vi "color.vi"() -> ()   [LabVIEW 2016]
uses:
  <vilib>/NXT/Subs/LVHSConnector.ctl
  <vilib>/NXT/LegoClasses/BrickReference/BrickReference.lvclass
  <vilib>/NXT/Block Support/NXT_InputPort.ctl
  <vilib>/NXT/Subs/ColorSensorColors.ctl
  <vilib>/NXT/Block Support/NXT_OutputPort.ctl
  <vilib>/NXT/Dual Mode Library/Display/drawNumber.vi
  <vilib>/NXT/Dual Mode Library/Sensors/Color_Detector.vi
  <vilib>/NXT/NXTIO Xnodes/NXTIONodeSubVIs/NXTStopMotors.vi
  <vilib>/NXT/NXTIO Xnodes/NXTIONodeSubVIs/NXTMoveMotors.vi
  <vilib>/NXT/NXTIO Xnodes/AddressXNode/NXTIOAddress.xnode
  <vilib>/NXT/NXTIO Xnodes/NXTIOXNode/NXTIO.xnode
panel:
  in  "NXT/EV3":T1
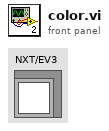
[diagram p1: front panel]
types:
  T1 = typedef "LVHSConnector.ctl" = refnum<class "BrickReference.lvclass">
  T2 = typedef "ColorSensorColors.ctl" = enum16{"No Color", "Black", "Blue", "Green", "Yellow", "Red", "White", "Brown"}
  T3 = typedef "NXT_OutputPort.ctl" = u8
  T4 = typedef "NXT_InputPort.ctl" = u32
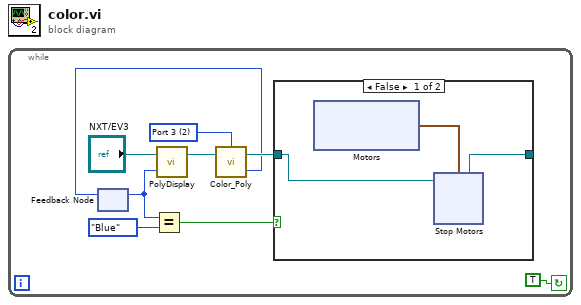
[diagram p0: block diagram]
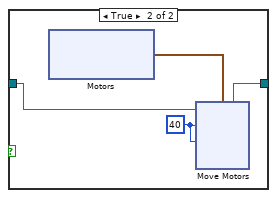
[diagram p2: hidden frame]
diagram:
  n1 = while {
    stop <- TRUE continue-if-true
    w9 = T4 2 items=["Port 1", "Port 2", "Port 3", "Port 4"] ("Port (Port 3)")
    n2 = feedback #1() -> (w2:T2)  [unwired: 1 in]
    n3 = Equal?(x=w2, y=ColorSensorColors."Blue") -> (x = y?=w7:bool)
    n4 = call-poly <vilib>:"PolyDisplay.vi"("number"=w2, "NXT/EV3"="NXT/EV3") -> ("NXT/EV3"=w4:T1)  [unwired: 2 in]
    n5 = call-poly <vilib>:"Color_Poly.vi"("NXT/EV3"=w4, "Port (Port 3)"=w9) -> ("Detected Color"=w3:T2, "NXT/EV3"=w6:T1)  [unwired: 1 in]
    n6 = feedback-in #1(w3) -> ()
    n7 = case shown="False" w7 {
      tunnel: w6 -> [w11 w22]
      tunnel: [w10 w20] -> _
      frame False {
        n8 = xnode "Motors"() -> ("Motor"=w12:cluster{"Port":T3, "Port":T3})
        n9 = xnode "Stop Motors"("Motors"=w12, "NXT/EV3"=w11) -> ("NXT/EV3"=w10:T1)
      }
      frame True {
        w19 = i8 40 ("Power/Speed 1")
        n10 = xnode "Motors"() -> ("Motor"=w21:cluster{"Port":T3, "Port":T3})
        n11 = xnode "Move Motors"("Power/Speed 2"=w19, "Power/Speed 1"=w19, "Motors"=w21, "NXT/EV3"=w22) -> ("NXT/EV3"=w20:T1)
      }
    }
  }
